vi "LVFunction_Imop_SlopesPostProcessor_Apply Substractor.vi"(0 "HasoSlopes in":refnum<class "HasoSlopes.lvclass">, 5 "HasoSlopes OUT":refnum<class "HasoSlopes.lvclass">, 7 "HasoSlopes to substract":refnum<class "HasoSlopes.lvclass">, 11 "error in (no error)":errorcluster) -> (4 "HasoSlopes out":refnum<class "HasoSlopes.lvclass">, 6 "HasoSlopes OUT 2":refnum<class "HasoSlopes.lvclass">, 15 "error out":errorcluster)   [LabVIEW 2020]
doc: "Subtracts Slopes_to_sutract to the input slopes.\n\n<B>Slopes_inIn</B> : HasoSlopes object, modified by the processor if Slopes_out = NULL.\n<B>Slopes_inOut</B> : HasoSlopes object, modified by the processor if Slopes_out = NULL.\n<B>Slopes_to_sutract</B> : HasoSlopes to subtract.\n<B>Slopes_out</B> : processed HasoSlopes object if not NULL."
uses:
  HasoSlopes.lvclass
  LVClass_HasoSlopes Read HasoSlopes _ property.vi
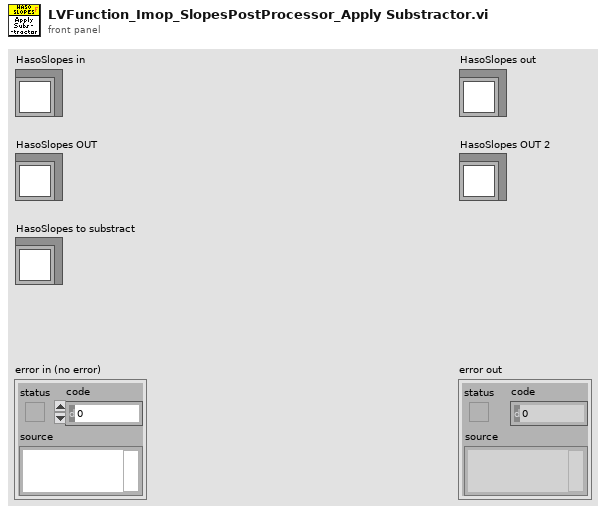
[diagram p1: front panel]
types:
  T1 = typedef "ClassID.ctl" = i64
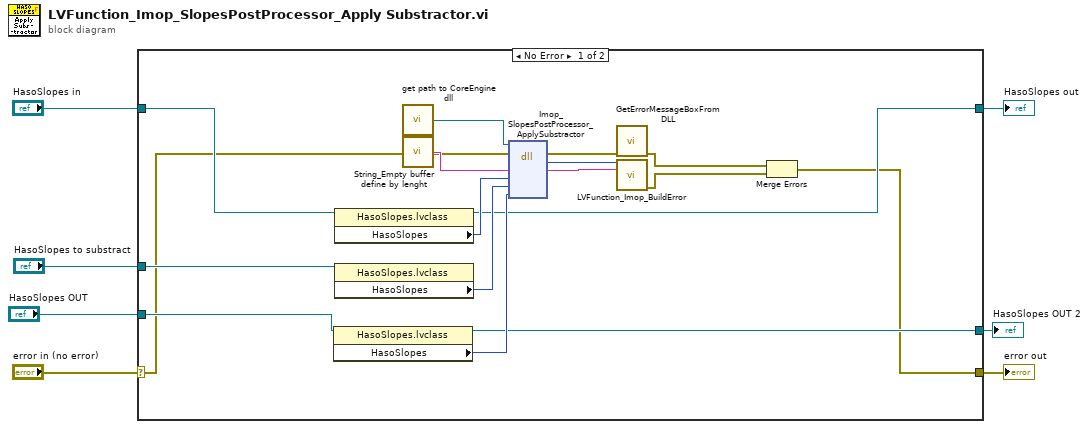
[diagram p0: block diagram]
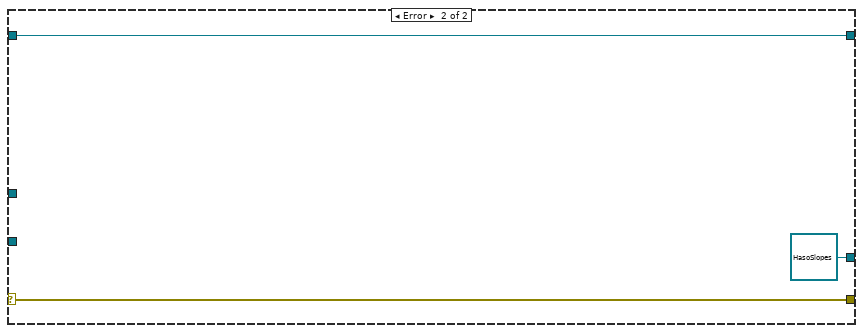
[diagram p2: hidden frame]
diagram:
  n1 = case shown="No Error" "error in (no error)" {
    selector: "error in (no error)" -> [w9 w27]
    tunnel: [w8 w27] -> w6
    tunnel: [w12 w26] -> w4
    tunnel: "HasoSlopes in" -> [w13 w26]
    tunnel: "HasoSlopes OUT" -> [w14 _]
    tunnel: "HasoSlopes to substract" -> [w11 _]
    tunnel: [w10 refnum<class "HasoSlopes.lvclass"> refnum ("HasoSlopes OUT")] -> w1
    frame No Error {
      n2 = property class="HasoSlopes.lvclass"(reference=w14) -> (reference out=w10:refnum<class "HasoSlopes.lvclass">, "HasoSlopes"=w15:T1)  [unwired: 1 in, 1 out]
      n3 = property class="HasoSlopes.lvclass"(reference=w13) -> (reference out=w12:refnum<class "HasoSlopes.lvclass">, "HasoSlopes"=w23:T1)  [unwired: 1 in, 1 out]
      n4 = property class="HasoSlopes.lvclass"(reference=w11) -> ("HasoSlopes"=w24:T1)  [unwired: 1 in, 2 out]
      n5 = call "get path to CoreEngine dll.vi"() -> ("path to wavekit library"=w18:path)  [unwired: 14 in, 1 out]
      n6 = call "String_Empty buffer define by lenght.vi"() -> ("Empty buffer"=w19:string)  [unwired: 1 in]
      n7 = dll-call lib="D:/FLE/0.Code/CoreEngine4_Suite/LV2011_interface/DLLs/c_interface_vc100.dll" fn="Imop_SlopesPostProcessor_ApplySubstractor"(path in=w18, error in=w9, "Message"=w19, "HasoSlopes IN"=w23, "HasoSlopes to substract"=w24, "HasoSlopes OUT"=w15) -> (error out=w22:errorcluster, "return type"=w20:i32, "Message"=w21:string)  [unwired: 4 in, 1 out]
      n8 = call "GetErrorMessageBoxFromDLL.vi"("error IN"=w22) -> ("error OUT"=w17:errorcluster)  [unwired: 10 in]
      n9 = call "LVFunction_Imop_BuildError.vi"("code"=w20, "String to Prepend to source (\"\")"=w21) -> ("error out"=w16:errorcluster)  [unwired: 13 in]
      n10 = Merge Errors(w17, w16) -> (w8:errorcluster)
    }
    frame Error {
    }
  }
  "error out" <- w6
  "HasoSlopes out" <- w4
  "HasoSlopes OUT 2" <- w1
